vi "MerweScSigPts_New_Default.vi"(11 "States":i32) -> (3 "MerweScaledSigmaPts":T1)   [LabVIEW 2019, in "Trajectory_Library.lvlib"]
doc: "Generates sigma points and weights according to Van der Merwe's 2004 dissertation[1] for the UnscentedKalmanFilter class.\n \nIt parametrizes the sigma points using alpha, beta, kappa terms, and is the version seen in most publications. Unless you know better, this should be your default choice.\n \nStates is the dimensionality of the state. 2*States+1 weights will be generated.\n \n[1] R. Van der Merwe \"Sigma-Point Kalman Filters for Probabilitic Inference in Dynamic State-Space Models\" (Doctoral dissertation)\n\nConstructs a generator for Van der Merwe scaled sigma points with default values for alpha, beta, and kappa.\n \nInputs:\n - states -- the number of states.\n\nOutputs:\n - MerweScaledSigmaPts -- data cluster"
uses:
  Trajectory_Library.lvlib
  MERWE_SCALED_SIGMA_PTS.ctl
  <vilib>/Analysis/Matrix/Datatypes/RealMatrix.ctl
  <vilib>/Analysis/Matrix/NI_Matrix.lvlib
panel:
  # "<?, 1>"
  # "<?, 1>"
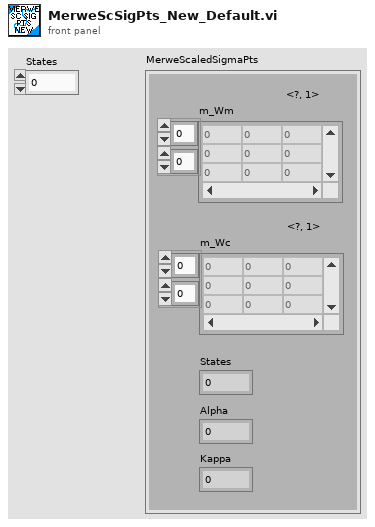
[diagram p1: front panel]
types:
  T1 = typedef "Trajectory_Library.lvlib/MERWE_SCALED_SIGMA_PTS.ctl" = cluster{"m_Wm":T2, "States":i32, "Alpha":dbl, "m_Wc":T2, "Kappa":i32}
  T2 = typedef "NI_Matrix.lvlib/RealMatrix.ctl" = dbl[][]
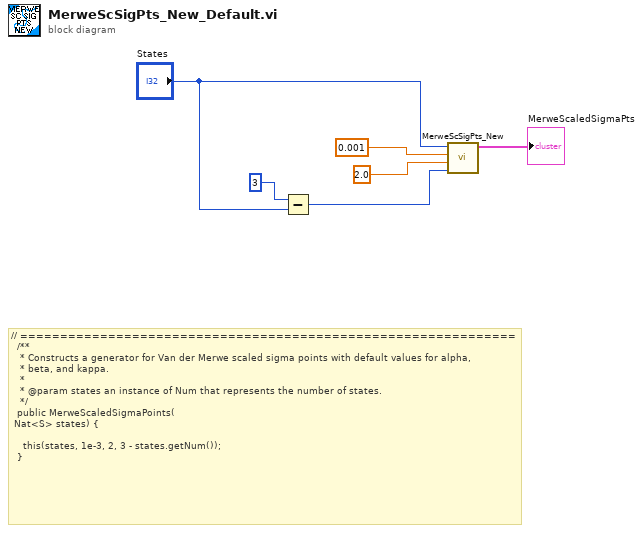
[diagram p0: block diagram]
diagram:
  # "// ==============================================================\n  /**\n   * Constructs a generator for Van der Merwe scaled sigma points with default values for alpha,\n   * beta, and kappa.\n   *\n   * @param states an instance of Num that represents the number of states.\n   */\n  public MerweScaledSigmaPoints(\n\tNat<S> states) {\n\n    this(states, 1e-3, 2, 3 - states.getNum());\n  }"
  n1 = Subtract(x=3, y="States") -> (x-y=w1:i32)
  n2 = call "MerweScSigPts_New.vi"("Kappa"=w1, "Beta"=2.0, "Alpha"=0.001, "States"="States") -> ("MerweScaledSigmaPts"=→"MerweScaledSigmaPts":T1)  [unwired: 7 in]
